vi "Wrap Positon.vi"(10 "Position":T2={"Point"={"X col"=0, "Y row"=0}, "Direction"=enum."Up (0x-1y)"}, 11 "Board":T1[][](array[typedef])) -> (2 "New X Col Out":i32, 3 "New Y Row Out":i32, 5 "Next Type Out":T1)   [LabVIEW 2020]
uses:
  Cluster_Position.ctl
  Cluster _Point.ctl
  ENUM_Direction.ctl
  RB ENUM_Board Space ID.ctl
  6d5c8255-a75b-4da9-b793-edfb9f72df74.vi
  7f198ed9-1c7b-480b-9577-486d82ee7cee.vi
  768c9844-8824-4fe2-84ad-4399243fc9c7.vi
  fa7c2455-60df-4803-901f-bc995bc2b9a5.vi
  <vilib>/Comparison/Equal/Equal Functor/Equal Functor.lvclass
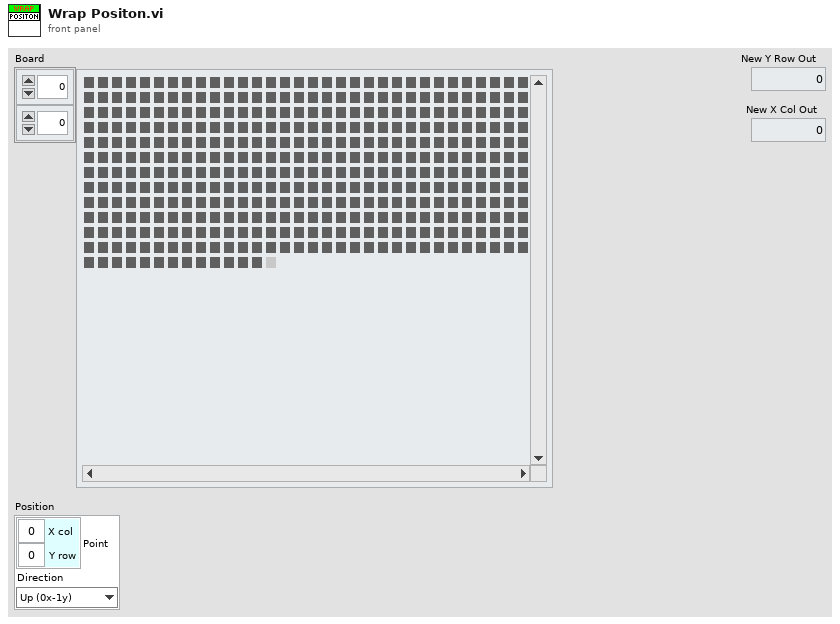
[diagram p1: front panel]
types:
  T1 = typedef "RB ENUM_Board Space ID.ctl" = enum32{"Blank", "Wall", "Tile", "Pos", "path"}
  T2 = typedef "Cluster_Position.ctl" = cluster{"Point":T3, "Direction":T4}
  T3 = typedef "Cluster _Point.ctl" = cluster{"X col":i32, "Y row":i32}
  T4 = typedef "ENUM_Direction.ctl" = enum16{"Right (1x0y)", "Down (0x1y)", "Left (-1x0y)]", "Up (0x-1y)"}
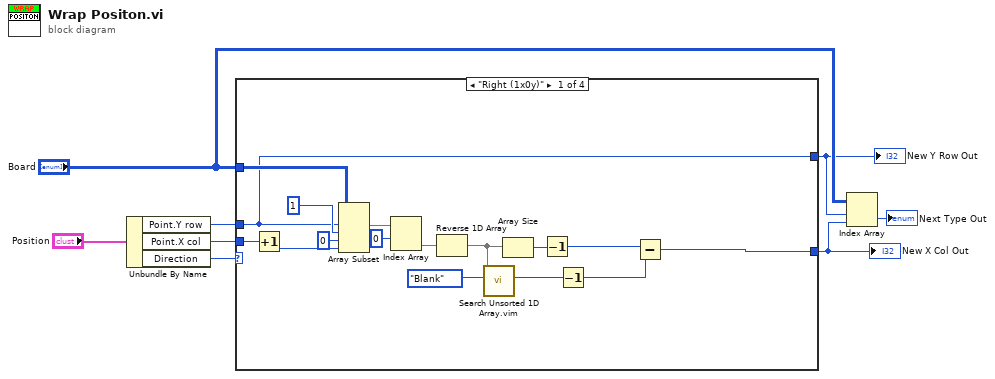
[diagram p0: block diagram]
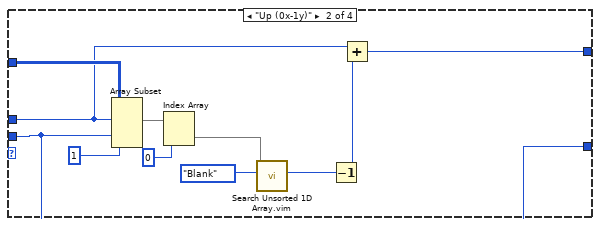
[diagram p2: hidden frame]
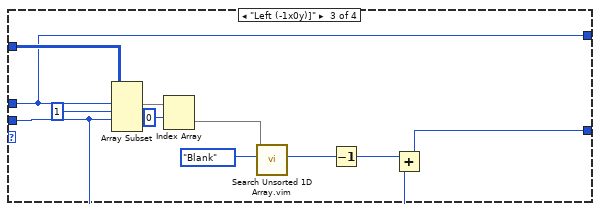
[diagram p3: hidden frame]
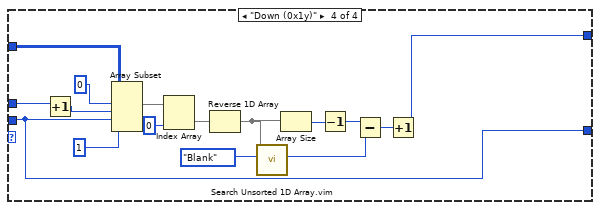
[diagram p4: hidden frame]
diagram:
  n1 = Unbundle By Name("Position") -> ("Point.Y row"=w6:i32, "Point.X col"=w5:i32, "Direction"=w7:T4)
  n2 = case shown="\"Right (1x0y)\"" w7 {
    tunnel: "Board" -> [w24 w35 w46 w62]
    tunnel: w6 -> [w9 w27 w39 w56]
    tunnel: [w9 w25 w39 w47] -> w3
    tunnel: [w11 w31 w37 w54] -> w2
    tunnel: w5 -> [w10 w31 w36 w54]
    frame "Right (1x0y)" {
      n3 = Increment(x=w10) -> (x+1=w12:i32)
      n4 = Array Subset(array=w24, index (row)=w9, length (row)=1 ("length"), index (col)=0 ("index"), length (col)=w12) -> (w23:T1[][])
      n5 = Index Array(array=w23, index (row)=0) -> (element=w21:T1[])  [unwired: 1 in]
      n6 = Reverse 1D Array(array=w21) -> (reversed array=w19:T1[])
      n7 = call "Search Unsorted 1D Array.vim"("element"=RB_ENUM_Board_Space_ID."Blank" ("Space"), "unsorted 1D array"=w19) -> ("index of element"=w16:i32)  [unwired: 9 in]
      n8 = Array Size(array=w19) -> (size(s)=w18:i32)
      n9 = Decrement(x=w18) -> (x-1=w17:i32)
      n10 = Decrement(x=w16) -> (x-1=w15:i32)
      n11 = Subtract(x=w17, y=w15) -> (x-y=w11:i32)
    }
    frame "Up (0x-1y)" {
      n12 = Array Subset(array=w35, index (row)=w27, index (col)=w31, length (col)=1 ("length")) -> (w34:T1[][])  [unwired: 1 in]
      n13 = Index Array(array=w34, index (col)=0 ("index (row)")) -> (element=w28:T1[])  [unwired: 1 in]
      n14 = call "Search Unsorted 1D Array.vim"("element"=RB_ENUM_Board_Space_ID."Blank" ("Space"), "unsorted 1D array"=w28) -> ("index of element"=w32:i32)  [unwired: 9 in]
      n15 = Decrement(x=w32) -> (x-1=w26:i32)
      n16 = Add(x=w27, y=w26) -> (x+y=w25:i32)
    }
    frame "Left (-1x0y)]" {
      n17 = Array Subset(array=w46, index (row)=w39, length (row)=1 ("length"), index (col)=w36) -> (w45:T1[][])  [unwired: 1 in]
      n18 = Index Array(array=w45, index (row)=0) -> (element=w42:T1[])  [unwired: 1 in]
      n19 = call "Search Unsorted 1D Array.vim"("element"=RB_ENUM_Board_Space_ID."Blank" ("Space"), "unsorted 1D array"=w42) -> ("index of element"=w43:i32)  [unwired: 9 in]
      n20 = Decrement(x=w43) -> (x-1=w40:i32)
      n21 = Add(x=w40, y=w36) -> (x+y=w37:i32)
    }
    frame "Down (0x1y)" {
      n22 = Increment(x=w56) -> (x+1=w55:i32)
      n23 = Array Subset(array=w62, index (row)=0 ("index"), length (row)=w55, index (col)=w54, length (col)=1 ("length")) -> (w61:T1[][])
      n24 = Index Array(array=w61, index (col)=0 ("disabled index (col)")) -> (element=w59:T1[])  [unwired: 1 in]
      n25 = Reverse 1D Array(array=w59) -> (reversed array=w52:T1[])
      n26 = call "Search Unsorted 1D Array.vim"("element"=RB_ENUM_Board_Space_ID."Blank" ("Space"), "unsorted 1D array"=w52) -> ("index of element"=w49:i32)  [unwired: 9 in]
      n27 = Array Size(array=w52) -> (size(s)=w51:i32)
      n28 = Decrement(x=w51) -> (x-1=w50:i32)
      n29 = Subtract(x=w50, y=w49) -> (x-y=w48:i32)
      n30 = Increment(x=w48) -> (x+1=w47:i32)
    }
  }
  "New X Col Out" <- w2
  "New Y Row Out" <- w3
  n31 = Index Array(array="Board", index (row)=w3, index (col)=w2) -> (element=→"Next Type Out":T1)
